vi "FlpLib InductorItoV 4.vi"(1 "L":sgl, 2 "dT":sgl, 7 "Current":sgl) -> (8 "Voltage":sgl)   [LabVIEW 2017]
uses:
  Calculus/Integrator/FlpLib Integrator 4.vi
  <userlib>/_NI FLP Library/FPGA/outsideSCTL/FlpLib Multiply Shared Instance 4.vi
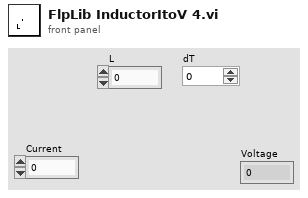
[diagram p1: front panel]
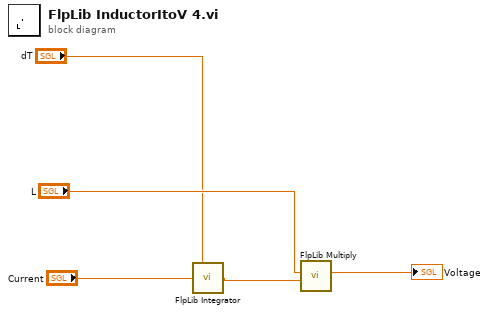
[diagram p0: block diagram]
diagram:
  n1 = call-poly "FlpLib Integrator.vi"("dt"="dT", "dx"="Current") -> ("x"=w2:sgl)  [unwired: 13 in]
  n2 = call-poly <userlib>:"FlpLib Multiply.vi"("y"=w2, "x"="L") -> ("x*y"=→"Voltage":sgl)  [unwired: 5 in]
